vi "ReHomeArms.vi"(11 "Array":bool[](array[boolean])) -> ()   [LabVIEW 2014]
uses:
  ReHomeLift.ctl
  <vilib>/Rock Robotics/WPI/CAN/TalonSRX/WPI_CANTalonSRX_APIControlMode.ctl
  <vilib>/Rock Robotics/WPI/CAN/TalonSRX/WPI_CANTalonSRX_APIFeedbackSelect.ctl
  Gantry/GantryGlobals.vi
panel:
  in  "Lift PID Gains":T1={"proportional gain (Kc)"=65.0, "integral time (Ti, min)"=0.0, "derivative time (Td, min)"=35.0}
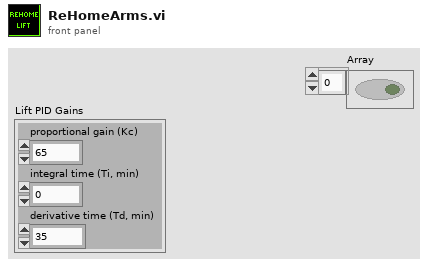
[diagram p1: front panel]
types:
  T1 = cluster{"proportional gain (Kc)":dbl, "integral time (Ti, min)":dbl, "derivative time (Td, min)":dbl}
  T2 = typedef "ReHomeLift.ctl" = enum16{"WaitingForInput", "ReHome"}
  T3 = typedef "WPI_CANTalonSRX_APIFeedbackSelect.ctl" = enum16{"Digital Quadrature Encoder", "Analog Potentiometer", "Analog Encoder"}
  T4 = typedef "WPI_CANTalonSRX_APIControlMode.ctl" = enum8{"Percent VBus", "Speed", "Position", "Slave", "Unchanged / Invalid"}
  T5 = typedef "WPI_MotorControlDeviceRef.ctl" = cluster{"DeviceStatus":errorcluster, "Type":T6, "PWM":cluster{"Controller":T7, "PWM Channel":T8, "DeadBand":T9}, "CAN":cluster{"Device Number":u8, "Control Mode":T10, "Semaphore":T11, "Max Vout":dbl, "TalonSRX Control Mode":T4}, "Invert":bool, "TransformRef":T12, "InvTransformRef":T12}
  T6 = typedef "WPI_MotorControlType.ctl" = enum16{"PWM", "CAN", "CANTalonSRX"}
  T7 = typedef "FPGA_TypedefDigitalModule.ctl" = enum16{"Controller 1"}
  T8 = typedef "FPGA_DIOPWMChannel.ctl" = enum8{"PWM 0", "PWM 1", "PWM 2", "PWM 3", "PWM 4", "PWM 5", "PWM 6", "PWM 7", "PWM 8", "PWM 9", "PWM MXP 0", "PWM MXP 1", "PWM MXP 2", "PWM MXP 3", "PWM MXP 4", "PWM MXP 5", "PWM MXP 6", "PWM MXP 7", "PWM MXP 8", "PWM MXP 9", "Invalid"}
  T9 = typedef "WPI_PWMDeadband.ctl" = cluster{"Name":string, "maxPositivePwm":i32, "minPositivePwm":i32, "centerPwm":i32, "maxNegativePwm":i32, "minNegativePwm":i32, "angularRange":u16}
  T10 = typedef "WPI_CANJaguar_ControlMode.ctl" = enum8{"Percent VBus", "Current", "Speed", "Position", "Voltage"}
  T11 = typedef "Semaphore RefNum" = refnum<k1>
  T12 = typedef "WPI_PWMTransform_ConPane.ctl" = refnum<vi>
  T13 = typedef "WPI_CANTalonSRX_GlobalStatus.ctl" = cluster{"Applied Throttle":dbl, "Module Enabled":bool, "CAN Error":errorcluster, "Closed Loop Error":dbl, "Forward Limit Switch Closed":bool, "Reverse Limit Switch Closed":bool, "Sensor Position":dbl, "Sensor Velocity":dbl, "Current":dbl, "Sticky Fault - Over Temp":bool, "Sticky Fault - Under Voltage":bool, "Sticky Fault - Forward Limit":bool, "Sticky Fault - Reverse Limit":bool, "Sticky Fault - Forward Soft Limit":bool, "Sticky Fault - Reverse Soft Limit":bool, "Brake is Enabled":bool, "Encoder Position":dbl, "Encoder Velocity":dbl, "Encoder Index Count":dbl, "Encoder A Pin State":bool, "Encoder B Pin State":bool, "Encoder Index Pin State":bool, "Analog In":dbl, "Analog In Velocity":dbl, "Temperature (C)":dbl, "Battery Voltage":dbl}
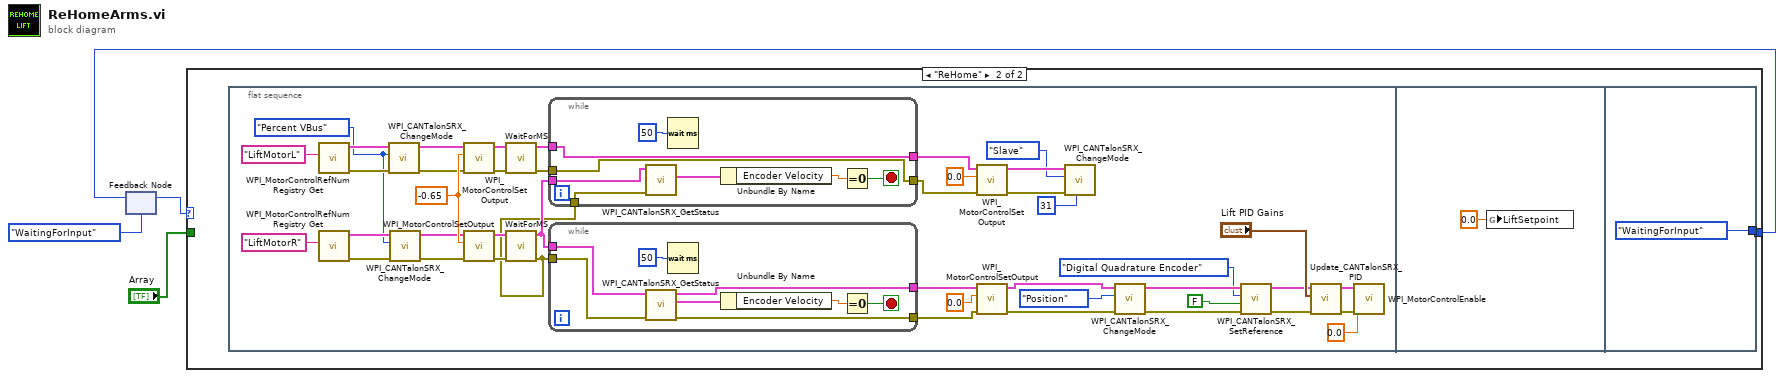
[diagram p0: block diagram]
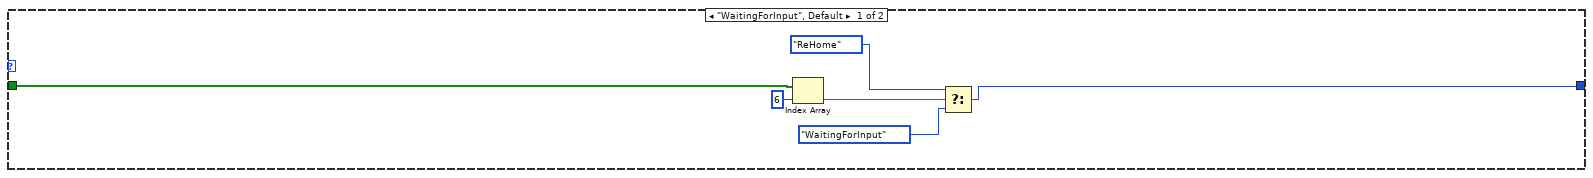
[diagram p2: hidden frame]
diagram:
  n1 = feedback #1(ReHomeLift."WaitingForInput" ("ReHome Lift")) -> (w3:T2)
  n2 = case shown="\"ReHome\"" w3 {
    tunnel: [w5 w11] -> w2
    tunnel: "Array" -> [w9 _]
    frame "WaitingForInput", Default {
      n3 = Index Array(array=w9, index=6) -> (element=w10:bool)
      n4 = Select(t=ReHomeLift."ReHome" ("ReHome Lift"), s=w10, f=ReHomeLift."WaitingForInput" ("ReHome Lift")) -> (s? t:f=w5:T2)
    }
    frame "ReHome" {
      n5 = flat-sequence {
        tunnel: [ReHomeLift."WaitingForInput" ("ReHome Lift")] -> w11
        frame #0 {
          w21 = WPI_CANTalonSRX_APIControlMode."Percent VBus" ("Control Mode")
          w53 = -0.65 ("Output")
          n6 = call <vilib>:"WPI_MotorControlRefNum Registry Get.vi"("refnum name"="LiftMotorL") -> ("error out"=w22:errorcluster, "MotorControlDevRef"=w23:T5)  [unwired: 9 in]
          n7 = call <vilib>:"WPI_MotorControlRefNum Registry Get.vi"("refnum name"="LiftMotorR") -> ("error out"=w24:errorcluster, "MotorControlDevRef"=w25:T5)  [unwired: 9 in]
          n8 = call <vilib>:"WPI_CANTalonSRX_ChangeMode.vi"("error in (no error)"=w22, "Control Mode"=w21, "CAN Talon SRX Ref"=w23) -> ("error out"=w13:errorcluster, "CAN Talon SRX Ref Out"=w14:T5)  [unwired: 7 in]
          n9 = call <vilib>:"WPI_CANTalonSRX_ChangeMode.vi"("error in (no error)"=w24, "Control Mode"=w21, "CAN Talon SRX Ref"=w25) -> ("error out"=w15:errorcluster, "CAN Talon SRX Ref Out"=w16:T5)  [unwired: 7 in]
          n10 = call <vilib>:"WPI_MotorControlSetOutput.vi"("error in (no error)"=w13, "Output"=w53, "MotorControlDevRef"=w14) -> ("error out"=w50:errorcluster, "MotorControlDevRef"=w51:T5)  [unwired: 6 in, 1 out]
          n11 = call <vilib>:"WPI_MotorControlSetOutput.vi"("error in (no error)"=w15, "Output"=w53, "MotorControlDevRef"=w16) -> ("error out"=w32:errorcluster, "MotorControlDevRef"=w33:T5)  [unwired: 6 in, 1 out]
          n12 = call "WaitForMS.vi"("error in"=w50, "MotorControlDevRef"=w51) -> ("error out"=w49:errorcluster, "MotorControlDevRef 2"=w48:T5)  [unwired: 8 in]
          n13 = call "WaitForMS.vi"("error in"=w32, "MotorControlDevRef"=w33) -> ("error out"=w30:errorcluster, "MotorControlDevRef 2"=w31:T5)  [unwired: 8 in]
          n14 = while {
            tunnel: w48 -> [w56]
            tunnel: w49 -> [w55]
            tunnel: w31 -> [w58]
            tunnel: w30 -> [w57]
            tunnel: [w56] -> w29
            tunnel: [w55] -> w28
            stop <- w59 stop-if-true
            n15 = call <vilib>:"WPI_CANTalonSRX_GetStatus.vi"("error in (no error)"=w57, "CAN Talon SRX Ref"=w58) -> ("Talon SRX Status"=w61:T13)  [unwired: 7 in, 2 out]
            n16 = Wait (ms)(milliseconds to wait=u32 50) -> ()  [unwired: 1 out]
            n17 = Unbundle By Name(w61) -> ("Encoder Velocity"=w60:dbl)
            n18 = Equal To 0?(x=w60) -> (x = 0?=w59:bool)
          }
          n19 = while {
            tunnel: w31 -> [w69]
            tunnel: w30 -> [w68]
            tunnel: [w65] -> w35
            tunnel: [w64] -> w34
            stop <- w63 stop-if-true
            n20 = call <vilib>:"WPI_CANTalonSRX_GetStatus.vi"("error in (no error)"=w68, "CAN Talon SRX Ref"=w69) -> ("error out"=w64:errorcluster, "Talon SRX Status"=w67:T13, "CAN Talon SRX Ref Out"=w65:T5)  [unwired: 7 in]
            n21 = Wait (ms)(milliseconds to wait=u32 50) -> ()  [unwired: 1 out]
            n22 = Unbundle By Name(w67) -> ("Encoder Velocity"=w66:dbl)
            n23 = Equal To 0?(x=w66) -> (x = 0?=w63:bool)
          }
          n24 = call <vilib>:"WPI_MotorControlSetOutput.vi"("error in (no error)"=w28, "Output"=0.0, "MotorControlDevRef"=w29) -> ("error out"=w20:errorcluster, "MotorControlDevRef"=w19:T5)  [unwired: 6 in, 1 out]
          n25 = call <vilib>:"WPI_MotorControlSetOutput.vi"("error in (no error)"=w34, "Output"=0.0, "MotorControlDevRef"=w35) -> ("error out"=w43:errorcluster, "MotorControlDevRef"=w44:T5)  [unwired: 6 in, 1 out]
          n26 = call <vilib>:"WPI_CANTalonSRX_ChangeMode.vi"("Master Device Number"=u8 31, "error in (no error)"=w20, "Control Mode"=WPI_CANTalonSRX_APIControlMode."Slave", "CAN Talon SRX Ref"=w19) -> ()  [unwired: 6 in, 2 out]
          n27 = call <vilib>:"WPI_CANTalonSRX_ChangeMode.vi"("error in (no error)"=w43, "Control Mode"=WPI_CANTalonSRX_APIControlMode."Position", "CAN Talon SRX Ref"=w44) -> ("error out"=w40:errorcluster, "CAN Talon SRX Ref Out"=w39:T5)  [unwired: 7 in]
          n28 = call <vilib>:"WPI_CANTalonSRX_SetReference.vi"("error in (no error)"=w40, "Reverse Feedback Sensor"=FALSE, "Feedback Reference"=WPI_CANTalonSRX_APIFeedbackSelect."Digital Quadrature Encoder", "CAN Talon SRX Ref"=w39) -> ("error out"=w37:errorcluster, "CAN Talon SRX Ref Out"=w38:T5)  [unwired: 6 in]
          n29 = call "Update_CANTalonSRX_PID.vi"("error in (no error)"=w37, "PID Gains"="Lift PID Gains", "CAN Talon SRX Ref"=w38) -> ("error out"=w41:errorcluster, "CAN Talon SRX Ref Out"=w42:T5)  [unwired: 7 in]
          n30 = call <vilib>:"WPI_MotorControlEnable.vi"("error in (no error)"=w41, "Encoder Initial Position"=0.0, "CAN Jaguar Ref"=w42) -> ()  [unwired: 7 in, 2 out]
        }
        frame #1 {
          n31 = global write "GantryGlobals.vi" "LiftSetpoint"(0.0 ("LiftSetpoint")) -> ()
        }
        frame #2 {
        }
      }
    }
  }
  n32 = feedback-in #1(w2) -> ()
